vi "01 - Syntax - Event API Syntax and Semantics.vi"() -> ()   [LabVIEW 2012]
panel:
  out "Tab Control":enum32{"Intro", "Join", "Links"}(tab)
  # "Jack Dunaway - CLA - LabVIEW Champion"
  # "Jack Dunaway - CLA - LabVIEW Champion"
  # "User Events Tips, Tricks, and Sundry"
  # "User Events Tips, Tricks, and Sundry"
  # "Follow along:"
  # "Follow along:"
  # "join.me/wirebirdlabs"
  # "join.me/wirebirdlabs"
  # "Download code:"
  # "Download code:"
  # "wirebird.co/CLA-Summit-2013-Paris"
  # "wirebird.co/CLA-Summit-2013-Paris"
  # "This Presentation\nhttp://wirebird.co/CLA-Summit-2013-Paris\n\nWirebird Labs\nhttps://wirebirdlabs.com"
  # "This Presentation\nhttp://wirebird.co/CLA-Summit-2013-Paris\n\nWirebird Labs\nhttps://wirebirdlabs.com"
  # "Links"
  # "Links"
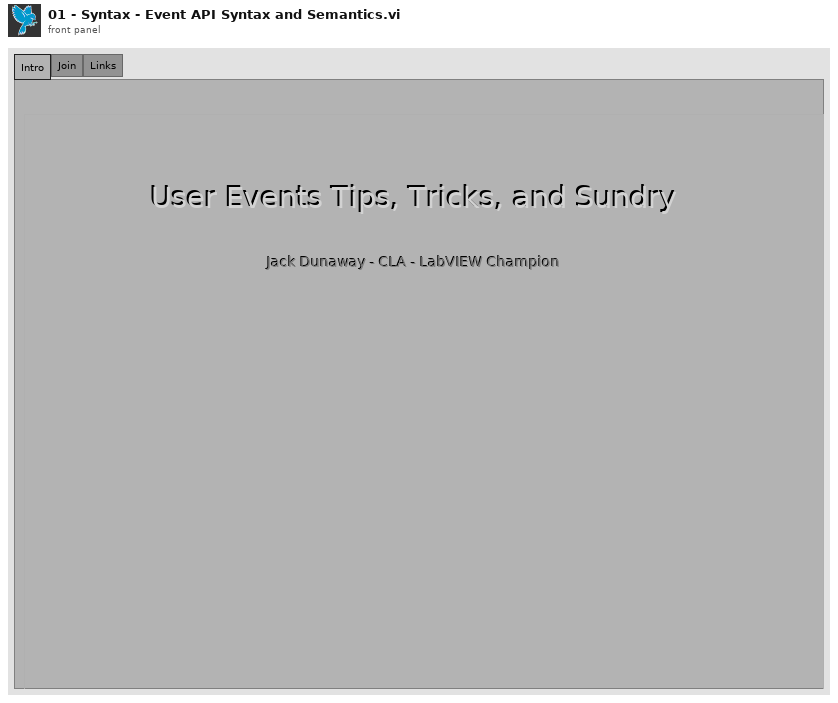
[diagram p1: front panel]
types:
  T1 = cluster{"Event Registration Refnum":refnum<event-registration>, "Event Registration Refnum":refnum<event-registration>}
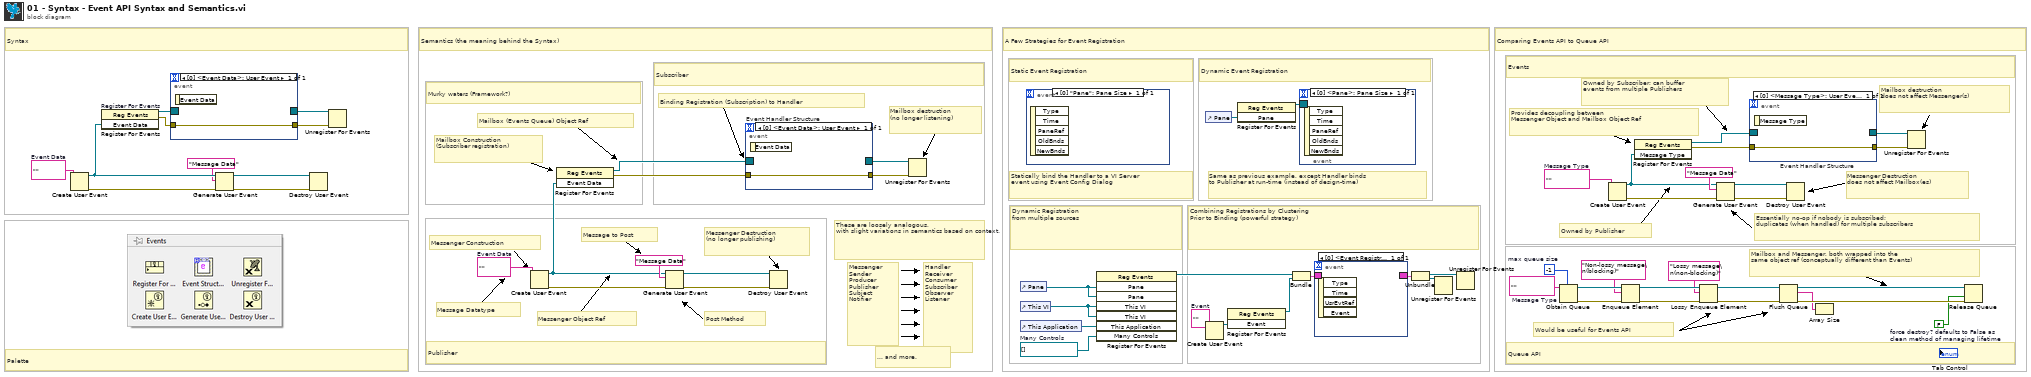
[diagram p0: block diagram]
diagram:
  w2 = -1  # max queue size
  w6 = refnum<vi>[] []  # Many Controls
  w10 = ""  # Event
  w17 = ""  # Message Type
  w20 = FALSE  # force destroy? defaults to False as clean method of managing lifetime
  w34 = ""  # Message Type
  w44 = ""  # Event Data
  w53 = ""  # Event Data
  # "These are loosely analogous,\nwith slight variations in semantics based on context."
  # "... and more."
  # "Combining Registrations by Clustering\nPrior to Binding (powerful strategy)"
  # "Dynamic Registration\nfrom multiple sources"
  # "Same as previous example, except Handler binds\nto Publisher at run-time (instead of design-time)"
  # "Dynamic Event Registration"
  # "Static Event Registration"
  # "A Few Strategies for Event Registration"
  # "Would be useful for Events API"
  # "Mailbox and Messenger, both wrapped into the\nsame object ref (conceptually different than Events)"
  # "Queue API"
  # "Events"
  # "Owned by Publisher"
  # "Comparing Events API to Queue API"
  # "Messenger Destruction\ndoes not affect Mailbox(es)"
  # "Mailbox destruction\ndoes not affect Messenger(s)"
  # "Essentially no-op if nobody is subscribed;\nduplicates (when handled) for multiple subscribers"
  # "Provides decoupling between\nMessenger Object and Mailbox Object Ref"
  # "Owned by Subscriber; can buffer\nevents from multiple Publishers"
  # "Messenger Object Ref"
  # "Message Datatype"
  # "Semantics (the meaning behind the Syntax)"
  # "Palette"
  # "Syntax"
  # "Messenger Destruction\n(no longer publishing)"
  # "Mailbox destruction\n(no longer listening)"
  # "Murky waters (Framework?)"
  # "Publisher"
  # "Subscriber"
  # "Post Method"
  # "Messenger Construction"
  # "Binding Registration (Subscription) to Handler"
  # "Handler\nReceiver\nConsumer\nSubscriber\nObserver\nListener"
  # "Messenger\nSender\nProducer\nPublisher\nSubject\nNotifier"
  # "Statically bind the Handler to a VI Server\nevent using Event Config Dialog"
  # "Mailbox Construction\n(Subscriber registration)"
  # "Message to Post"
  # "Mailbox (Events Queue) Object Ref"
  n1 = Create User Event(user event datatype=w53) -> (user event=w57:refnum<user-event>, error out=w54:errorcluster)  [unwired: 1 in]
  n2 = register-events "Register For Events"(w57) -> (reference out=w58:refnum<event-registration>, error out=w51:errorcluster)  [unwired: 2 in]
  n3 = event shown="[0] <Event Data>: User Event" {
    selector: w58 -> [_]
    dyn-events: [_] -> w52
    timeout: _ -> [_]
    tunnel: w51 -> [w59]
    tunnel: [w59] -> w50
    event User Event {
      n4 = event-data() -> ()  [unwired: 1 in, 1 out]
    }
  }
  n5 = Generate User Event(user event=w57, event data cluster="Message Data" ("event data"), error in=w54) -> (user event out=w56:refnum<user-event>, error out=w55:errorcluster)
  n6 = Destroy User Event(user event=w56, error in=w55) -> ()  [unwired: 1 out]
  n7 = Unregister For Events(event registration refnum=w52, error in=w50) -> ()  [unwired: 1 out]
  n8 = Create User Event(user event datatype=w44) -> (user event=w40:refnum<user-event>, error out=w43:errorcluster)  [unwired: 1 in]
  n9 = register-events(w40) -> (reference out=w39:refnum<event-registration>, error out=w46:errorcluster)  [unwired: 2 in]
  n10 = Generate User Event(user event=w40, event data cluster="Message Data" ("event data"), error in=w43) -> (user event out=w41:refnum<user-event>, error out=w42:errorcluster)
  n11 = event "Event Handler Structure" shown="[0] <Event Data>: User Event" {
    selector: w39 -> [_]
    dyn-events: [_] -> w45
    timeout: _ -> [_]
    tunnel: w46 -> [w60]
    tunnel: [w60] -> w47
    event User Event {
      n12 = event-data() -> ()  [unwired: 1 in, 1 out]
    }
  }
  n13 = Destroy User Event(user event=w41, error in=w42) -> ()  [unwired: 1 out]
  n14 = Unregister For Events(event registration refnum=w45, error in=w47) -> ()  [unwired: 1 out]
  n15 = control-ref of="Pane"() -> (w14:refnum<vi>)
  n16 = control-ref of="This VI"() -> (w13:refnum<vi>)
  n17 = control-ref of="This Application"() -> (w12:refnum<vi>)
  n18 = event shown="[0] \"Pane\": Pane Size" {
    selector: _ -> [_]
    dyn-events: _ -> [_]
    timeout: _ -> [_]
    event Pane Size {
      n19 = event-data() -> ()  [unwired: 1 in, 5 out]
    }
  }
  n20 = register-events(w14, w14, w13, w13, w12, w6) -> (reference out=w9:refnum<event-registration>)  [unwired: 2 in, 1 out]
  n21 = control-ref of="Pane"() -> (w15:refnum<vi>)
  n22 = Create User Event(user event datatype=w10) -> (user event=w11:refnum<user-event>)  [unwired: 1 in, 1 out]
  n23 = register-events(w11) -> (reference out=w8:refnum<event-registration>)  [unwired: 2 in, 1 out]
  n24 = register-events(w15) -> (reference out=w16:refnum<event-registration>)  [unwired: 2 in, 1 out]
  n25 = Bundle("Event Registration Refnum"=w9, "Event Registration Refnum"=w8) -> (w7:T1)  [unwired: 1 in]
  n26 = event shown="[0] <Pane>: Pane Size" {
    selector: w16 -> [_]
    dyn-events: _ -> [_]
    timeout: _ -> [_]
    event Pane Size {
      n27 = event-data() -> ()  [unwired: 1 in, 5 out]
    }
  }
  n28 = event shown="[0] <Event Registration Refnum.Event>: User Event" {
    selector: w7 -> [_]
    dyn-events: [_] -> w5
    timeout: _ -> [_]
    event User Event {
      n29 = event-data() -> ()  [unwired: 1 in, 4 out]
    }
  }
  n30 = Unbundle(w5) -> ("Event Registration Refnum"=w3:refnum<event-registration>, "Event Registration Refnum"=w4:refnum<event-registration>)
  n31 = Unregister For Events(event registration refnum=w4) -> ()  [unwired: 1 in, 1 out]
  n32 = Unregister For Events(event registration refnum=w3) -> ()  [unwired: 1 in, 1 out]
  n33 = Obtain Queue(max queue size (-1, unlimited)=w2, element data type=w17) -> (queue out=w28:refnum<queue>, error out=w27:errorcluster)  [unwired: 3 in, 1 out]
  n34 = Create User Event(user event datatype=w34) -> (user event=w30:refnum<user-event>, error out=w33:errorcluster)  [unwired: 1 in]
  n35 = Enqueue Element(queue=w28, element="Non-lossy message\n(blocking)", error in (no error)=w27) -> (queue out=w26:refnum<queue>, error out=w25:errorcluster)  [unwired: 1 in, 1 out]
  n36 = register-events(w30) -> (reference out=w29:refnum<event-registration>, error out=w36:errorcluster)  [unwired: 2 in]
  n37 = Lossy Enqueue Element(queue=w26, element="Lossy message\n(non-blocking)", error in (no error)=w25) -> (queue out=w23:refnum<queue>, error out=w24:errorcluster)  [unwired: 2 out]
  n38 = Generate User Event(user event=w30, event data cluster="Message Data" ("event data"), error in=w33) -> (user event out=w31:refnum<user-event>, error out=w32:errorcluster)
  n39 = event "Event Handler Structure" shown="[0] <Message Type>: User Event" {
    selector: w29 -> [_]
    dyn-events: [_] -> w35
    timeout: _ -> [_]
    tunnel: w36 -> [w61]
    tunnel: [w61] -> w37
    event User Event {
      n40 = event-data() -> ()  [unwired: 1 in, 1 out]
    }
  }
  n41 = Flush Queue(queue=w23, error in (no error)=w24) -> (queue out=w22:refnum<queue>, remaining elements=w1:string[], error out=w21:errorcluster)
  n42 = Destroy User Event(user event=w31, error in=w32) -> ()  [unwired: 1 out]
  n43 = Array Size(array=w1) -> ()  [unwired: 1 out]
  n44 = Unregister For Events(event registration refnum=w35, error in=w37) -> ()  [unwired: 1 out]
  n45 = Release Queue(queue=w22, force destroy? (F)=w20, error in (no error)=w21) -> ()  [unwired: 3 out]
